vi "Set Default.vi"(8 "error in (no error)":errorcluster, 11 "DMM Config Msg in":refnum<class "DMM List Triggers Msg.lvclass">) -> (0 "error out":errorcluster, 3 "DMM Config Msg out":refnum<class "DMM List Triggers Msg.lvclass">)   [LabVIEW 2020, in "DMM Msg.lvlib" / "DMM List Triggers Msg.lvclass"]
doc: "Restore private data to a defined default state.\n\nThis implementation sets:\nAwait reply, -1ms timeout at normal priority without publish"
uses:
  DMM List Triggers Msg.lvclass
  PPL/HDH.Actor Framework.Core.Actor.lvlibp/1abvi3w/vi.lib/ActorFramework/Message Enqueuer/Message Priority.ctl
  PPL/HDH.Actor Framework.Core.Publisher.lvlibp/Messages/Response Msg/Response Core/Controls/Ctl_SendFunction.ctl
  DMM Msg/DMM Msg.lvclass
  PPL/HDH.Actor Framework.Core.Instrument Handler.lvlibp/Messages/Instrument Msg/Instrument Msg.lvclass
  PPL/HDH.Actor Framework.Core.Publisher.lvlibp
  PPL/HDH.Actor Framework.Core.Actor.lvlibp/1abvi3w/vi.lib/ActorFramework/Message Enqueuer/Message Enqueuer.lvclass
  C:/Current projects/WS/PPL/HDH.Actor Framework.Core.Instrument Handler.lvlibp/Messages/Instrument Msg/Instrument Msg.lvclass
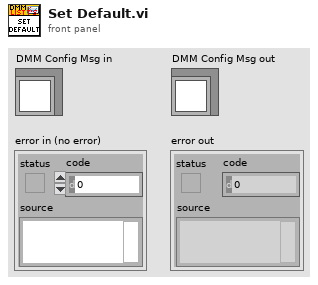
[diagram p1: front panel]
types:
  T1 = typedef "HDH.Actor Framework.Core.Publisher.lvlibp/Ctl_SendFunction.ctl" = enum16{"Send and Forget", "Request Reply", "Await Reply"}
  T2 = typedef "HDH.Actor Framework.Core.Actor.lvlibp/Message Enqueuer.lvclass/Message Priority.ctl" = enum16{"Low", "Normal", "High"}
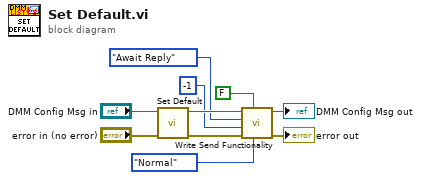
[diagram p0: block diagram]
diagram:
  n1 = call-parent "Set Default.vi"("error in (no error)"="error in (no error)", "Flex Msg in"="DMM Config Msg in") -> ("error out"=w5:errorcluster, "Flex Msg out"=w10:refnum<class "DMM List Triggers Msg.lvclass">)  [unwired: 8 in]
  n2 = call "Write Send Functionality.vi"("Message Priority(Normal)"=Message_Priority."Normal", "Publish Data?(T)"=FALSE, "error in (no error)"=w5, "Timeout if Waiting(-1ms)"=-1, "Send Function(Await Reply)"=Ctl_SendFunction."Await Reply", "Instrument Msg in"=w10) -> ("error out"=→"error out":errorcluster, "Instrument Msg out"=→"DMM Config Msg out":refnum<class "DMM List Triggers Msg.lvclass">)  [unwired: 4 in]
